vi "SimulationDataAnalysis.vi"() -> ()   [LabVIEW 2018]
uses:
  General Libraries/Photon Filtering.lvlib
panel:
  out "mask":dbl[][](graph)
  out "FFT":dbl[][](graph)
  out "sum FFT":dbl
  in  "Intensity Graph 2":dbl[][](graph)=array1280x960[1228800 elements]
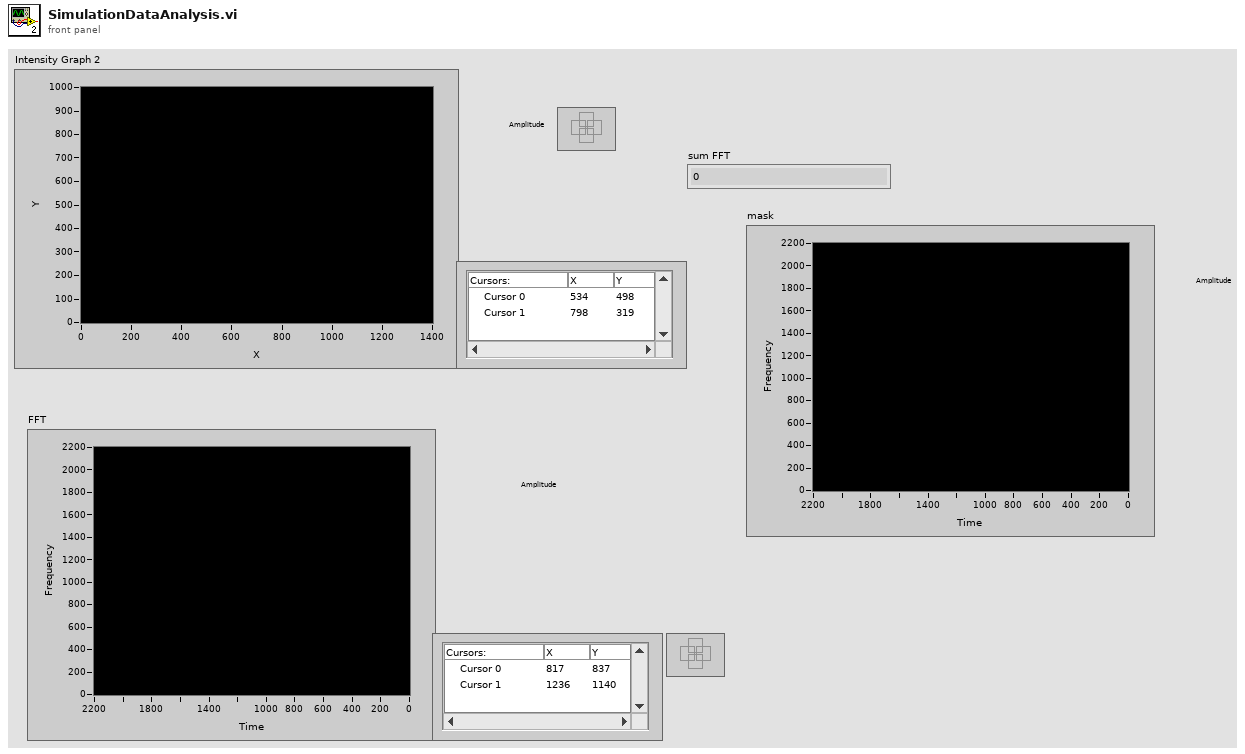
[diagram p1: front panel]
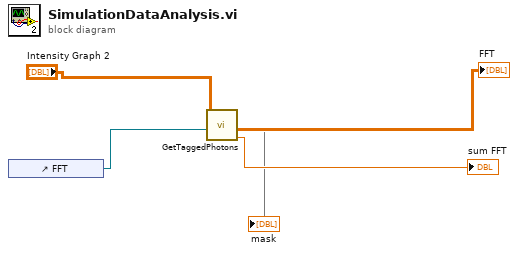
[diagram p0: block diagram]
diagram:
  n1 = control-ref of="FFT"() -> (w2:refnum<vi>)
  n2 = call "GetTaggedPhotons.vi"("FFT reference"=w2, "double precision float"="Intensity Graph 2") -> ("FFT full energy"=→"sum FFT":dbl, "FFT modulous"=→"FFT":dbl[][], 6:→"mask")  [unwired: 5 in, 2 out]
